vi "Prober_MoveToXYZTheta.vi"(6 "Theta location [mdeg]":string="none", 7 "ProbeStationControl in":refnum<class "ProbeStationControl.lvclass">, 8 "error in (no error)":errorcluster, 9 "Z location [µm]":string="none", 10 "Y location [µm]":string="none", 11 "X location [µm]":string="none") -> (0 "error out":errorcluster, 2 "String":string, 3 "ProbeStationControl out":refnum<class "ProbeStationControl.lvclass">)   [LabVIEW 2013, in "ProbeStationControl.lvclass"]
uses:
  ProbeStationControl.lvclass
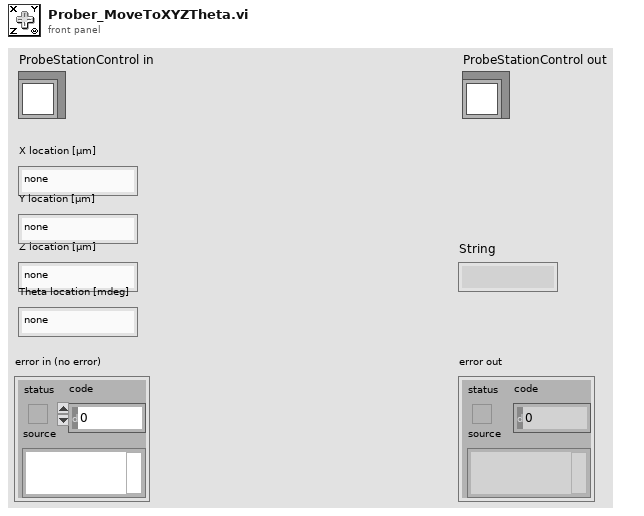
[diagram p1: front panel]
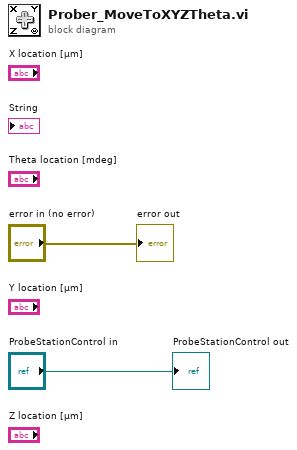
[diagram p0: block diagram]
diagram:
  "error out" <- "error in (no error)"
  "ProbeStationControl out" <- "ProbeStationControl in"
